vi "get_volt_meas_set_array.vi"(9 "DAQmx Device Name":tag="Dev1") -> (1 "Voltage meas settings array":T1[](array[typedef]) {"Terminal Configuration" items=["default"=-1, "RSE"=10083, "NRSE"=10078, "Differential"=10106, "Pseudodifferential"=12529]})   [LabVIEW 2023]
doc: "Creates an array of voltage measurement setups of\n- Measure Vin\n- Measure VRsense\n- Measure Vout"
uses:
  ctl_voltage_meas_settings_cluster.ctl
  ctl_volt_meas_modes_enum.ctl
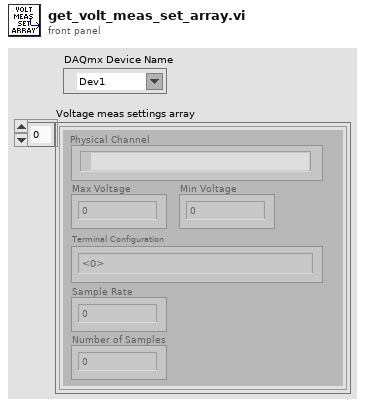
[diagram p1: front panel]
types:
  T1 = typedef "ctl_voltage_meas_settings_cluster.ctl" = cluster{"Physical Channel":tag, "Min Voltage":dbl, "Max Voltage":dbl, "Terminal Configuration":i32, "Sample Rate":dbl, "Number of Samples":i32}
  T2 = typedef "ctl_volt_meas_modes_enum.ctl" = enum16{"Measure Vin", "Measure VRsense", "Measure Vout"}
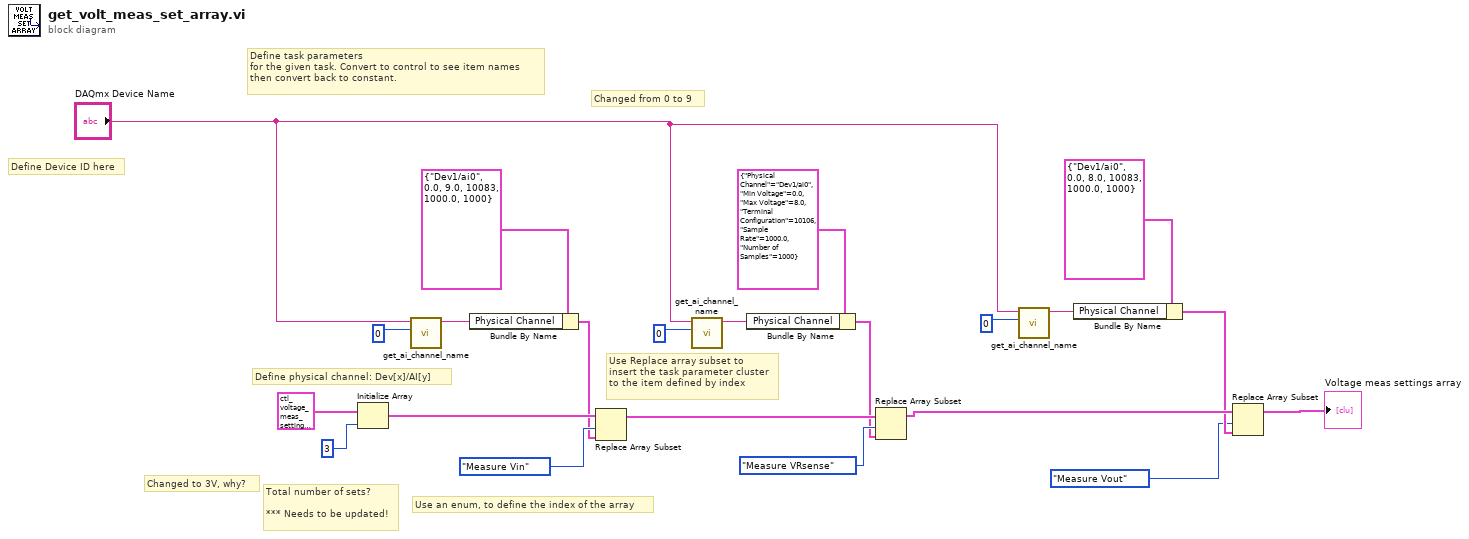
[diagram p0: block diagram]
diagram:
  # "Changed to 3V, why?"
  # "Changed from 0 to 9"
  # "Use an enum, to define the index of the array"
  # "Use Replace array subset to\ninsert the task parameter cluster\nto the item defined by index"
  # "Define physical channel: Dev[x]/AI[y]"
  # "Define task parameters\nfor the given task. Convert to control to see item names\nthen convert back to constant."
  # "Define Device ID here"
  # "Total number of sets?\n\n*** Needs to be updated!"
  n1 = Initialize Array(T1 {"Physical Channel"="Dev1/ai0", "Min Voltage"=-5.0, "Max Voltage"=5.0, "Terminal Configuration"=-1, "Sample Rate"=1000.0, "Number of Samples"=100} ("Voltage meas settings"), 3 ("dimension size")) -> (w17:T1[])
  n2 = call "get_ai_channel_name.vi"("AI number"=i8 0 ("input 2"), "DAQmx Device Name"="DAQmx Device Name") -> ("DAQmx Physical Channel"=w13:tag)  [unwired: 9 in]
  n3 = Bundle By Name(cluster=T1 {"Physical Channel"="Dev1/ai0", "Min Voltage"=0.0, "Max Voltage"=9.0, "Terminal Configuration"=10083, "Sample Rate"=1000.0, "Number of Samples"=1000} ("Voltage meas settings"), "Physical Channel"=w13) -> (w15:T1)
  n4 = Replace Array Subset(array=w17, new element=w15, index=ctl_volt_meas_modes_enum."Measure Vin" ("Voltage meas modes")) -> (w18:T1[])
  n5 = call "get_ai_channel_name.vi"("AI number"=i8 0 ("input 2"), "DAQmx Device Name"="DAQmx Device Name") -> ("DAQmx Physical Channel"=w10:tag)  [unwired: 9 in]
  n6 = Bundle By Name(cluster=T1 {"Physical Channel"="Dev1/ai0", "Min Voltage"=0.0, "Max Voltage"=8.0, "Terminal Configuration"=10106, "Sample Rate"=1000.0, "Number of Samples"=1000} ("Voltage meas settings"), "Physical Channel"=w10) -> (w9:T1)
  n7 = Replace Array Subset(array=w18, new element=w9, index=ctl_volt_meas_modes_enum."Measure VRsense" ("Voltage meas modes")) -> (w4:T1[])
  n8 = call "get_ai_channel_name.vi"("AI number"=i8 0 ("input 2"), "DAQmx Device Name"="DAQmx Device Name") -> ("DAQmx Physical Channel"=w6:tag)  [unwired: 9 in]
  n9 = Bundle By Name(cluster=T1 {"Physical Channel"="Dev1/ai0", "Min Voltage"=0.0, "Max Voltage"=8.0, "Terminal Configuration"=10083, "Sample Rate"=1000.0, "Number of Samples"=1000} ("Voltage meas settings"), "Physical Channel"=w6) -> (w2:T1)
  n10 = Replace Array Subset(array=w4, new element=w2, index=ctl_volt_meas_modes_enum."Measure Vout" ("Voltage meas modes")) -> (→"Voltage meas settings array":T1[])
